vi "COD质控流程 (子VI).vi"(10 "CODMn量程切换":enum32{"H", "L", "AUTO"}(ring)=enum."AUTO", 11 "COD":bool) -> (2 "CODMn中断报警":bool, 3 "布尔":bool)   [LabVIEW 2016, in "质控单元.lvlib"]
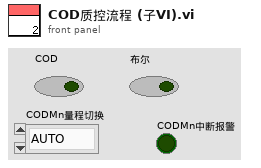
[diagram p1: front panel]
types:
  T1 = enum16{"待机", "启动水样测量", "水样测量中", "启动加标", "启动加标回收", "加标回收测量中", "结束"}
  T2 = cluster{"测量模式":enum16{"水样测量", "标样核查", "零点核查", "跨度核查", "空白测试", "加标回收", "平行样", "校零", "校标"}}
  T3 = enum16{"空闲", "水样测试", "标样核查", "零点核查", "跨度核查", "空白测试", "平行样测试", "质控样", "空白校准", "标样校准", "加标回收"}
  T4 = enum16{"空闲", "水样测试", "标样核查", "零点核查", "跨度核查", "空白测试", "平行样测试", "加标回收", "空白校准", "标样校准", "初始化（清洗）"}
  T5 = cluster{"量程":dbl, "检出限":dbl, "加标前水样浓度":dbl, "加标后水样浓度":dbl, "加标水杯定容体积":dbl, "加标母液浓度":dbl, "加标体积":dbl, "加标回收率":dbl}
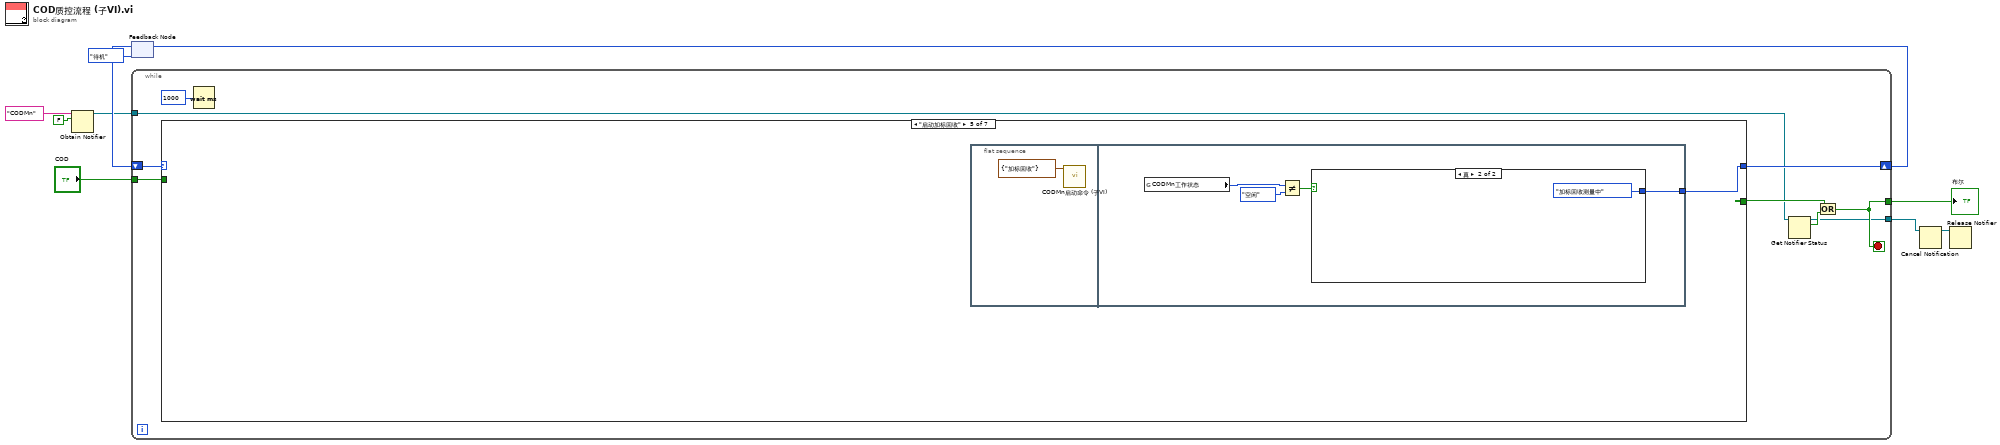
[diagram p0: block diagram]
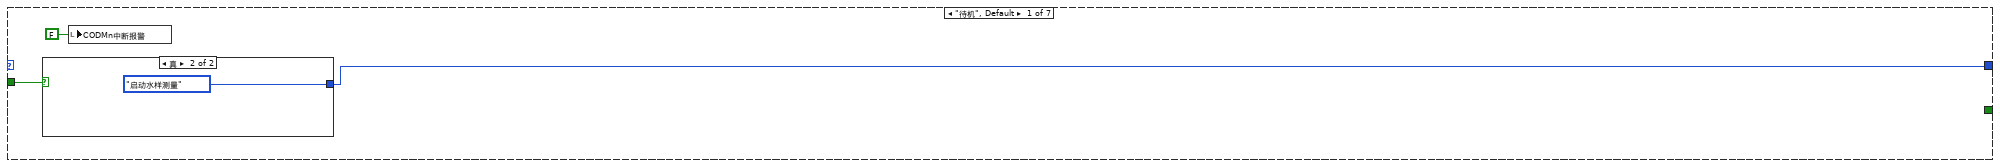
[diagram p2: hidden frame]
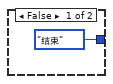
[diagram p3: hidden frame]
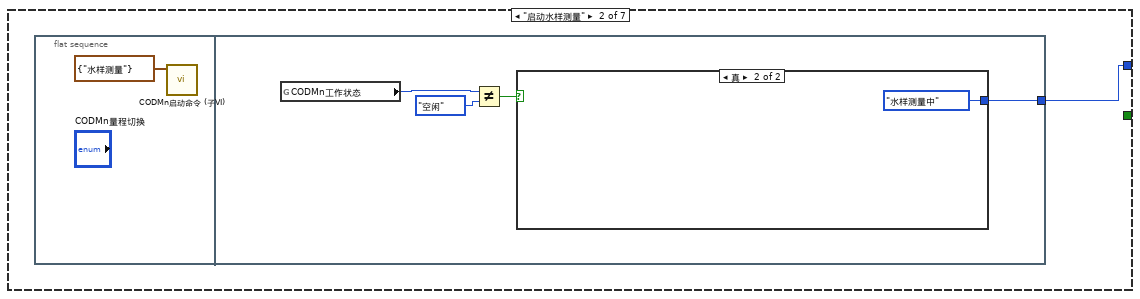
[diagram p4: hidden frame]
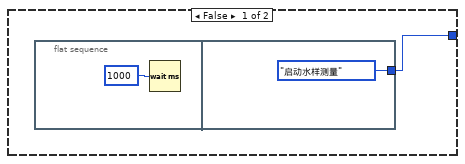
[diagram p5: hidden frame]
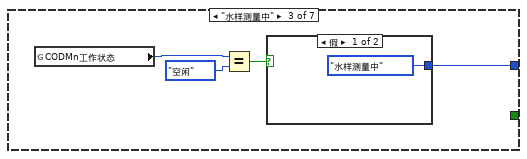
[diagram p6: hidden frame]
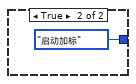
[diagram p7: hidden frame]
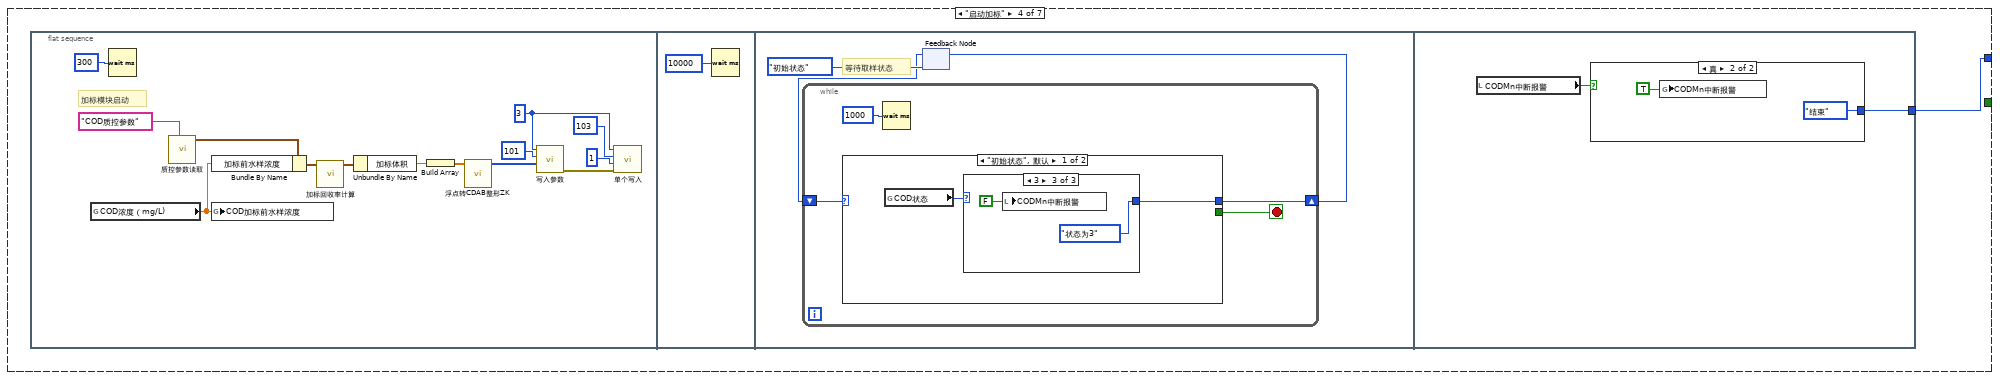
[diagram p8: hidden frame]
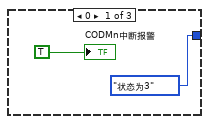
[diagram p9: hidden frame]
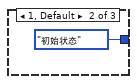
[diagram p10: hidden frame]
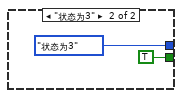
[diagram p11: hidden frame]
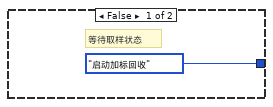
[diagram p12: hidden frame]
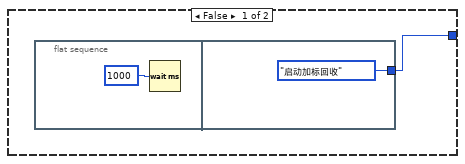
[diagram p13: hidden frame]
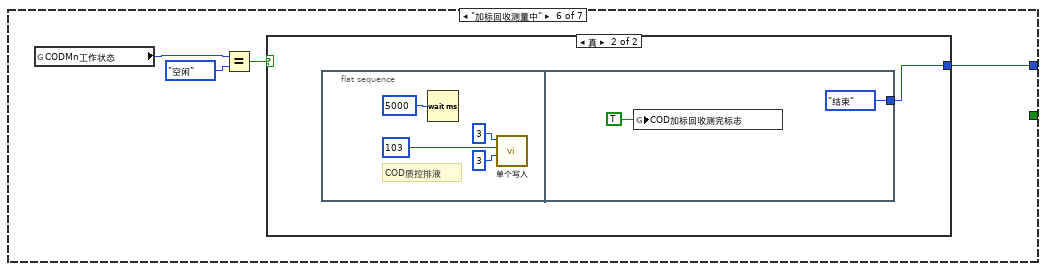
[diagram p14: hidden frame]
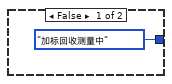
[diagram p15: hidden frame]
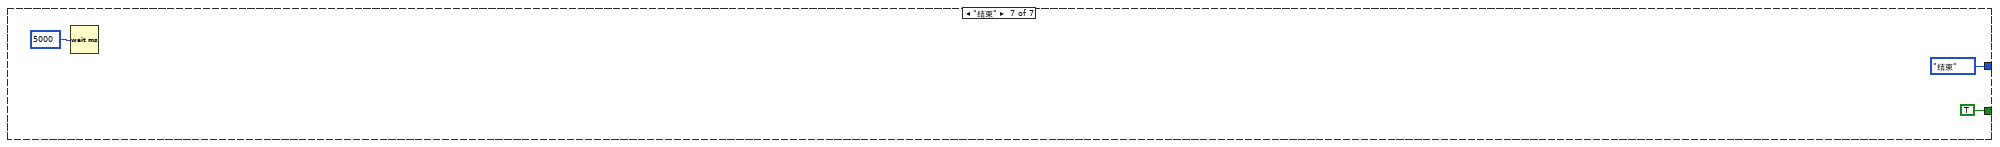
[diagram p16: hidden frame]
diagram:
  n1 = Obtain Notifier(name (unnamed)="CODMn" ("名称（未命名）"), notification data type=FALSE) -> (notifier out=w3:refnum<notifier>)  [unwired: 2 in, 2 out]
  n2 = feedback #1(T1."待机") -> (w6:T1)
  n3 = while {
    tunnel: "COD" -> [w19]
    tunnel: [w13] -> w8
    shift-right: [w18] -> w9
    shift-left: w6 -> [w17]
    tunnel: w3 -> [w12]
    tunnel: [w11] -> w1
    stop <- w13 stop-if-true
    n4 = case shown="\"启动加标回收\"" w17 {
      tunnel: [w22 w25 w38 w41 w78 w91 T1."结束"] -> w18
      tunnel: [_ _ _ _ _ _ TRUE] -> w14
      tunnel: w19 -> [w21 _ _ _ _ _ _]
      frame "待机", Default {
        n5 = case shown="真" w21 {
          tunnel: [T1."结束" T1."启动水样测量"] -> w22
          frame False {
          }
          frame True {
          }
        }
        n6 = local write "CODMn中断报警"(FALSE ("CODMn中断报警")) -> ()
      }
      frame "启动水样测量" {
        n7 = flat-sequence {
          tunnel: [w30] -> w25
          frame #0 {
            n8 = call "CODMn启动命令 (子VI).vi"("启动测量模式"=T2 {"测量模式"=enum."水样测量"}) -> ()  [unwired: 10 in, 1 out]
          }
          frame #1 {
            n9 = global read "与CODMn交互全局.vi" "CODMn工作状态"() -> (w29:T4)
            n10 = Not Equal?(x=w29, y=T3."空闲") -> (x != y?=w27:bool)
            n11 = case shown="真" w27 {
              tunnel: [w31 T1."水样测量中"] -> w30
              frame False {
                n12 = flat-sequence {
                  tunnel: [T1."启动水样测量"] -> w31
                  frame #0 {
                    n13 = Wait (ms)(milliseconds to wait=u32 1000 ("等待时间（毫秒）")) -> ()  [unwired: 1 out]
                  }
                  frame #1 {
                  }
                }
              }
              frame True {
              }
            }
          }
        }
      }
      frame "水样测量中" {
        n14 = global read "与CODMn交互全局.vi" "CODMn工作状态"() -> (w37:T4)
        n15 = Equal?(x=w37, y=T3."空闲") -> (x = y?=w35:bool)
        n16 = case shown="假" w35 {
          tunnel: [T1."水样测量中" T1."启动加标"] -> w38
          frame False {
          }
          frame True {
          }
        }
      }
      frame "启动加标" {
        n17 = flat-sequence {
          tunnel: [w74] -> w41
          frame #0 {
            w43 = u16 3 ("value")
            # "加标模块启动"
            n18 = global read "与CODMn交互全局.vi" "COD浓度（mg/L)"() -> (w44:dbl)
            n19 = Wait (ms)(milliseconds to wait=u32 300 ("等待时间（毫秒）")) -> ()  [unwired: 1 out]
            n20 = call "质控参数读取.vi"("section"="COD质控参数") -> ("参数"=w53:T5)  [unwired: 9 in, 1 out]
            n21 = Bundle By Name(cluster=w53, "加标前水样浓度"=w44) -> (w54:T5)
            n22 = global write "水样浓度全局.vi" "COD加标前水样浓度"(w44) -> ()
            n23 = call "加标回收率计算.vi"("参数"=w54) -> ("参数 out"=w52:T5)  [unwired: 9 in, 1 out]
            n24 = Unbundle By Name(w52) -> ("加标体积"=w45:dbl)
            n25 = Build Array(w45) -> (w51:dbl[])
            n26 = call "浮点转CDAB整形ZK.vi"("浮点数"=w51) -> ("CDAB整形输出"=w46:u16[])  [unwired: 10 in]
            n27 = call "写入参数.vi"("values"=w46, "starting address"=u16 101, "Slave ID"=w43) -> ("error out"=w50:errorcluster)  [unwired: 8 in]
            n28 = call "单个写入.vi"("Error in"=w50, "value"=u16 1, "address"=u16 103, "Slave ID"=w43) -> ()  [unwired: 7 in, 1 out]
          }
          frame #1 {
            n29 = Wait (ms)(milliseconds to wait=u32 10000 ("等待时间（毫秒）")) -> ()  [unwired: 1 out]
          }
          frame #2 {
            # "等待取样状态"
            n30 = feedback #2(enum16{"初始状态", "状态为3"}."初始状态") -> (w58:enum16{"初始状态", "状态为3"})
            n31 = while {
              shift-right: [w62] -> w57
              shift-left: w58 -> [w63]
              stop <- w61 stop-if-true
              n32 = case shown="\"初始状态\", 默认" w63 {
                tunnel: [w65 enum16{"初始状态", "状态为3"}."状态为3"] -> w62
                tunnel: [_ TRUE] -> w61
                frame "初始状态", Default {
                  n33 = global read "加标回收状态全局变量.vi" "COD状态"() -> (w64:u16)
                  n34 = case shown="3" w64 {
                    tunnel: [enum16{"初始状态", "状态为3"}."状态为3" enum16{"初始状态", "状态为3"}."初始状态" enum16{"初始状态", "状态为3"}."状态为3"] -> w65
                    frame 0 {
                      "CODMn中断报警" <- TRUE ("CODMn中断报警")
                    }
                    frame 1, Default {
                    }
                    frame 3 {
                      n35 = local write "CODMn中断报警"(FALSE ("CODMn中断报警")) -> ()
                    }
                  }
                }
                frame "状态为3" {
                }
              }
              n36 = Wait (ms)(milliseconds to wait=u32 1000 ("等待时间（毫秒）")) -> ()  [unwired: 1 out]
            }
            n37 = feedback-in #2(w57) -> ()
          }
          frame #3 {
            n38 = local read "CODMn中断报警"() -> (w73:bool)
            n39 = case shown="真" w73 {
              tunnel: [T1."启动加标回收" T1."结束"] -> w74
              frame False {
                # "等待取样状态"
              }
              frame True {
                n40 = global write "质控中断报警全局.vi" "CODMn中断报警"(TRUE ("CODMn中断报警")) -> ()
              }
            }
          }
        }
      }
      frame "启动加标回收" {
        n41 = flat-sequence {
          tunnel: [w83] -> w78
          frame #0 {
            n42 = call "CODMn启动命令 (子VI).vi"("启动测量模式"=T2 {"测量模式"=enum."加标回收"}) -> ()  [unwired: 10 in, 1 out]
          }
          frame #1 {
            n43 = global read "与CODMn交互全局.vi" "CODMn工作状态"() -> (w82:T4)
            n44 = Not Equal?(x=w82, y=T3."空闲") -> (x != y?=w80:bool)
            n45 = case shown="真" w80 {
              tunnel: [w84 T1."加标回收测量中"] -> w83
              frame False {
                n46 = flat-sequence {
                  tunnel: [T1."启动加标回收"] -> w84
                  frame #0 {
                    n47 = Wait (ms)(milliseconds to wait=u32 1000 ("等待时间（毫秒）")) -> ()  [unwired: 1 out]
                  }
                  frame #1 {
                  }
                }
              }
              frame True {
              }
            }
          }
        }
      }
      frame "加标回收测量中" {
        n48 = global read "与CODMn交互全局.vi" "CODMn工作状态"() -> (w90:T4)
        n49 = Equal?(x=w90, y=T3."空闲") -> (x = y?=w88:bool)
        n50 = case shown="真" w88 {
          tunnel: [T1."加标回收测量中" w93] -> w91
          frame False {
          }
          frame True {
            n51 = flat-sequence {
              tunnel: [T1."结束"] -> w93
              frame #0 {
                # "COD质控排液"
                n52 = Wait (ms)(milliseconds to wait=u32 5000 ("等待时间（毫秒）")) -> ()  [unwired: 1 out]
                n53 = call "单个写入.vi"("value"=u16 3, "address"=u16 103, "Slave ID"=u8 3) -> ()  [unwired: 8 in, 1 out]
              }
              frame #1 {
                n54 = global write "质控测完标志全局 1.vi" "COD加标回收测完标志"(TRUE ("COD加标回收测完标志")) -> ()
              }
            }
          }
        }
      }
      frame "结束" {
        n55 = Wait (ms)(milliseconds to wait=u32 5000 ("等待时间（毫秒）")) -> ()  [unwired: 1 out]
      }
    }
    n56 = Wait (ms)(milliseconds to wait=u32 1000 ("等待时间（毫秒）")) -> ()  [unwired: 1 out]
    n57 = Get Notifier Status(notifier=w12) -> (notifier out=w11:refnum<notifier>, current notification=w15:bool)  [unwired: 1 in, 3 out]
    n58 = Or(x=w14, y=w15) -> (x .or. y?=w13:bool)
  }
  "布尔" <- w8
  n59 = feedback-in #1(w9) -> ()
  n60 = Cancel Notification(0:w1) -> (8:w2:refnum<notifier>)  [unwired: 1 in, 2 out]
  n61 = Release Notifier(notifier=w2) -> ()  [unwired: 2 in, 3 out]
